vi "SeqMap_Write.vi"(8 "error in (no error)":errorcluster, 10 "Value":variant, 11 "Tag":string) -> (0 "error out":errorcluster)   [LabVIEW 2016, in "SeqProcessor.lvlib"]
uses:
  SeqProcessor.lvlib
  <vilib>/addons/PointValueMap/subVIs/Point_Write_variant.vi
  <vilib>/addons/PointValueMap/PointValueMap.lvlib
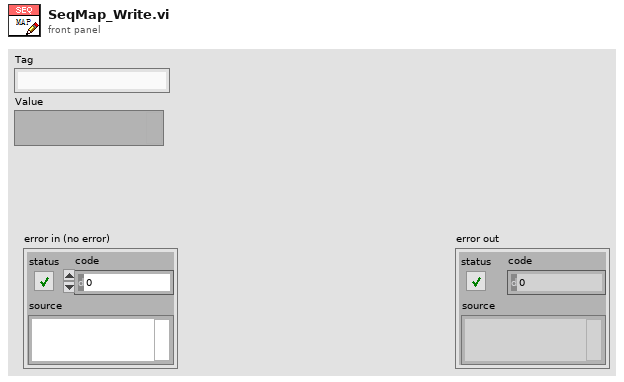
[diagram p1: front panel]
types:
  T1 = typedef "PointValueMap.lvlib/PointMap.ctl" = refnum<data-value>
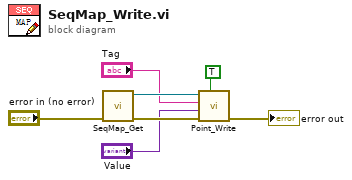
[diagram p0: block diagram]
diagram:
  n1 = call "SeqMap_Get.vi"("error in (no error)"="error in (no error)") -> ("error out"=w6:errorcluster, "SeqMap"=w5:T1)  [unwired: 9 in]
  n2 = call-poly <vilib>:"Point_Write.vi"("Auto Create?"=TRUE, "Error In"=w6, "Value"="Value", "Tag"="Tag", "Map"=w5) -> ("Error Out"=→"error out":errorcluster)  [unwired: 5 in, 1 out]
